vi "operacja.vi"(11 "Array in":dbl[](array[numeric])) -> (2 "Array out":dbl[](array[numeric]), 3 "Numeric":dbl)   [LabVIEW 2016]
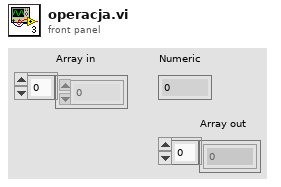
[diagram p1: front panel]
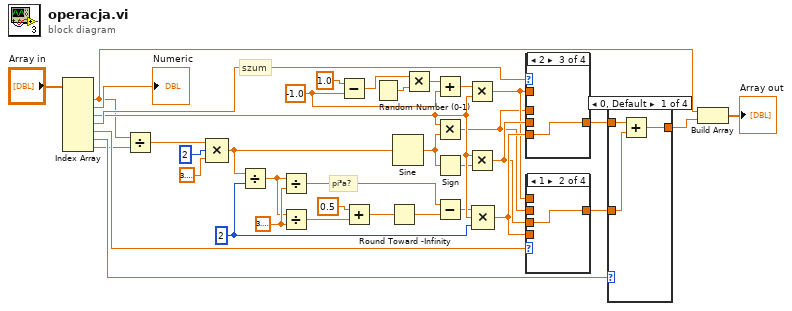
[diagram p0: block diagram]
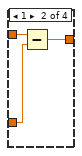
[diagram p2: hidden frame]
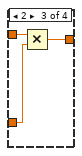
[diagram p3: hidden frame]
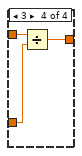
[diagram p4: hidden frame]
diagram:
  w1 = 2
  w23 = 3.141592653589793
  w11 = -1.0 ("x")
  # "pi³a?"
  # "szum"
  n1 = Index Array(array="Array in") -> (element #1=w8:dbl, element #2=→"Numeric":dbl, element #3=w34:dbl, element #4=w35:dbl, element #5=w36:dbl, element #6=w37:dbl, element #7=w7:dbl)  [unwired: 7 in]
  n2 = Divide(x=w8, y=w7) -> (x/y=w6:dbl)
  n3 = Compound Arithmetic op=MULTIPLY(w6, 2, 3.141592653589793) -> (w2:dbl)
  n4 = Divide(x=w2, y=w1) -> (x/y=w3:dbl)
  n5 = Divide(x=w3, y=w23) -> (x/y=w24:dbl)
  n6 = Divide(x=w3, y=w23) -> (x/y=w27:dbl)
  n7 = Subtract(x=1.0, y=w11) -> (x-y=w13:dbl)
  n8 = Add(x=0.5, y=w27) -> (x+y=w26:dbl)
  n9 = Random Number (0-1)() -> (number: 0 to 1=w14:dbl)
  n10 = Round Toward -Infinity(1:w26) -> (0:w25:dbl)
  n11 = Sine(x=w2) -> (sin(x)=w19:dbl)
  n12 = Multiply(x=w13, y=w14) -> (x*y=w15:dbl)
  n13 = Add(x=w15, y=w11) -> (x+y=w16:dbl)
  n14 = Multiply(x=w34, y=w19) -> (x*y=w17:dbl)
  n15 = Sign(1:w19) -> (0:w20:dbl)
  n16 = Subtract(x=w24, y=w25) -> (x-y=w28:dbl)
  n17 = Multiply(x=w16, y=w34) -> (x*y=w18:dbl)
  n18 = Multiply(x=w34, y=w20) -> (x*y=w21:dbl)
  n19 = Compound Arithmetic op=MULTIPLY(w28, w34, w1) -> (w29:dbl)
  n20 = case shown="2" w35 {
    tunnel: w17 -> [w38 _ _ _]
    tunnel: w21 -> [_ w39 _ _]
    tunnel: w29 -> [_ _ w40 _]
    tunnel: w18 -> [_ _ _ w41]
    tunnel: [w38 w39 w40 w41] -> w9
    frame 0, Default {
    }
    frame 1 {
    }
    frame 2 {
    }
    frame 3 {
    }
  }
  n21 = case shown="1" w36 {
    tunnel: w17 -> [w42 _ _ _]
    tunnel: w21 -> [_ w43 _ _]
    tunnel: w29 -> [_ _ w44 _]
    tunnel: w18 -> [_ _ _ w45]
    tunnel: [w42 w43 w44 w45] -> w10
    frame 0, Default {
    }
    frame 1 {
    }
    frame 2 {
    }
    frame 3 {
    }
  }
  n22 = case shown="0, Default" w37 {
    tunnel: w9 -> [w48 w51 w54 w57]
    tunnel: w10 -> [w47 w50 w53 w56]
    tunnel: [w46 w49 w52 w55] -> w30
    frame 0, Default {
      n23 = Add(x=w48, y=w47) -> (x+y=w46:dbl)
    }
    frame 1 {
      n24 = Subtract(x=w51, y=w50) -> (x-y=w49:dbl)
    }
    frame 2 {
      n25 = Multiply(x=w54, y=w53) -> (x*y=w52:dbl)
    }
    frame 3 {
      n26 = Divide(x=w57, y=w56) -> (x/y=w55:dbl)
    }
  }
  n27 = Build Array(w8, w30) -> (→"Array out":dbl[])
